vi "Convert Data.vi"(8 "error in":errorcluster, 10 "refnum to write":refnum<file>, 11 "refnum to read":refnum<file>) -> (0 "error out":errorcluster, 2 "refnum to write 2":refnum<file>, 3 "refnum to read 2":refnum<file>)   [LabVIEW 2017]
uses:
  <vilib>/Analysis/polynomials.llb/Polynomial Roots (DBL).vi
  <vilib>/Analysis/NI_AALPro.lvlib
  <vilib>/Analysis/NI_AALBase.lvlib
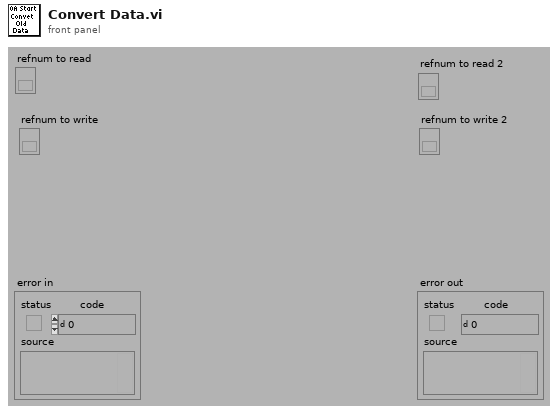
[diagram p1: front panel]
types:
  T1 = cluster{"name":string, "multiplier":sgl, "offset":sgl, "sensor sensitivity (mV/EU)":dbl, "engineering units":enum16{"custom...", "V", "Pa", "g", "m/s^2", "m/s", "m", "in/s^2", "in/s", "in"}}[]
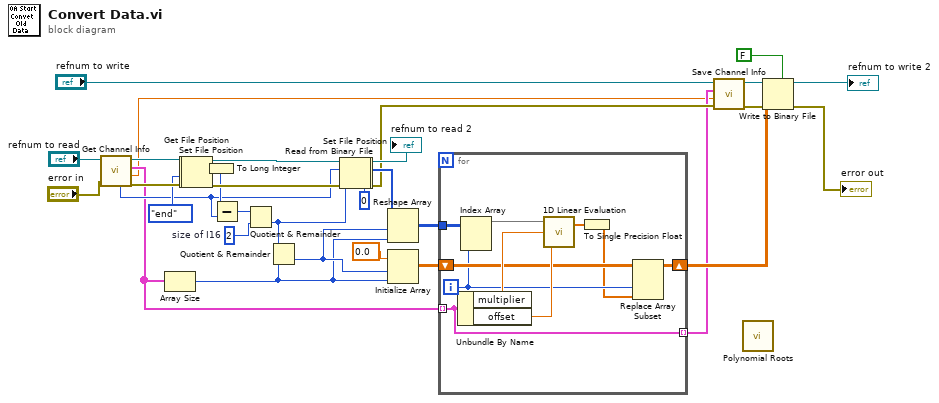
[diagram p0: block diagram]
diagram:
  w28 = 2  # size of I16
  n1 = call <vilib>:"Get Channel Info.vi"("error in"="error in", "refnum in"="refnum to read") -> ("error out"=w32:errorcluster, "time"=w7:dbl, "channel information"=w9:T1, "dup refnum"=w33:refnum<file>, "data offset"=w26:i32)  [unwired: 4 in, 1 out]
  n2 = Array Size(array=w9) -> (size(s)=w20:i32)
  n3 = Set File Position(refnum=w33, from (0:start)=enum16{"start", "end", "current"}."end" ("pos mode (0:2)"), error in=w32) -> (refnum out=w3:refnum<file>, error out=w2:errorcluster)  [unwired: 1 in]
  n4 = Get File Position(4:w2, 7:w3) -> (0:w35:errorcluster, 2:w1:i64, 3:w34:refnum<file>)
  n5 = To Long Integer(number=w1) -> (32bit integer=w30:i32)
  n6 = Subtract(x=w30, y=w26) -> (x-y=w29:i32)
  n7 = Quotient & Remainder(x=w29, y=w28) -> (floor(x/y)=w27:i32)  [unwired: 1 out]
  n8 = Quotient & Remainder(x=w27, y=w20) -> (floor(x/y)=w21:i32)  [unwired: 1 out]
  n9 = Set File Position(offset (in bytes) (0)=w26, refnum=w34, error in=w35) -> (refnum out=w5:refnum<file>, error out=w4:errorcluster)  [unwired: 1 in]
  n10 = Read from Binary File(5:i16 0, 8:w4, 10:w27, 11:w5) -> (0:w11:errorcluster, 2:w23:i16[], 3:→"refnum to read 2":refnum<file>)  [unwired: 2 in, 1 out]
  n11 = Reshape Array(w23, w21, w20) -> (w22:i16[][])
  n12 = Initialize Array(sgl 0.0 ("element"), w21, w20) -> (w18:sgl[][])
  n13 = for {
    tunnel: w22 -> [w46]
    tunnel: w9 -> [w37] mode=indexing
    shift-right: [w38] -> w17
    shift-left: w18 -> [w41]
    tunnel: [w37] -> w8 mode=indexing
    i -> [w40]
    n14 = Unbundle By Name(w37) -> ("multiplier"=w44:sgl, "offset"=w43:sgl)
    n15 = Index Array(array=w46, index (col)=w40) -> (element=w45:i16[])  [unwired: 1 in]
    n16 = call <vilib>:"1D Linear Evaluation.vi"("offset"=w43, "scale"=w44, "X"=w45) -> ("Y[i]=X[i]*a+b"=w42:dbl[])  [unwired: 1 out]
    n17 = To Single Precision Float(number=w42) -> (single precision float=w39:sgl[])
    n18 = Replace Array Subset(array=w41, new element=w39, index (col)=w40) -> (w38:sgl[][])  [unwired: 1 in]
  }
  n19 = call <vilib>:"Save Channel Info.vi"("error in"=w11, "time"=w7, "channel info"=w8, "refnum in"="refnum to write") -> ("error out"=w14:errorcluster, "refnum out"=w15:refnum<file>)  [unwired: 6 in]
  n20 = call-poly <vilib>:"Polynomial Roots.vi"() -> ()  [unwired: 10 in, 2 out]
  n21 = Write to Binary File(file (use dialog)=w15, data=w17, error in=w14, 5:FALSE ("prepend array or string size? (T)")) -> (refnum out=→"refnum to write 2":refnum<file>, error out=→"error out":errorcluster)  [unwired: 2 in, 1 out]
